vi "Drive to Distance.vi"(9 "Acceptable Error (in)":dbl, 10 "Target in Inches":dbl) -> (2 "Complete?":bool)   [LabVIEW 2020]
uses:
  Global Sensor Reads.vi
  <vilib>/Rock Robotics/WPI/RobotDrive/WPI_RobotDriveArcadeDrive_Standard(NoSaturation).vi
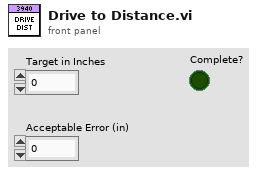
[diagram p1: front panel]
types:
  T1 = typedef "WPI_RobotDriveDevRef.ctl" = cluster{"DevStatus":errorcluster, "Motors[]":T2[], "Square Inputs":bool, "Max Output":dbl}
  T2 = typedef "WPI_MotorControlDeviceRef.ctl" = cluster{"DeviceStatus":errorcluster, "Type":T3, "PWM":cluster{"PWM Channel":T4, "DeadBand":T5}, "CAN":cluster{"Device Number":u8, "SetOutput VI Ref":variant, "GetOutput VI Ref":variant, "Enable VI Ref":variant, "Disable VI Ref":variant, "Data":variant}, "Invert":bool, "DIO PWM":cluster{"PWM \"Enable\" Channel":T4, "DIOChannel":T6, "PWM Rate":dbl}}
  T3 = typedef "WPI_MotorControlType.ctl" = enum16{"PWM", "CAN", "DIO PWM"}
  T4 = typedef "FPGA_DIOPWMChannel.ctl" = enum8{"PWM 0", "PWM 1", "PWM 2", "PWM 3", "PWM 4", "PWM 5", "PWM 6", "PWM 7", "PWM 8", "PWM 9", "PWM MXP 0", "PWM MXP 1", "PWM MXP 2", "PWM MXP 3", "PWM MXP 4", "PWM MXP 5", "PWM MXP 6", "PWM MXP 7", "PWM MXP 8", "PWM MXP 9", "Invalid"}
  T5 = typedef "WPI_PWMDeadband.ctl" = cluster{"Name":string, "maxPositivePwm":i32, "minPositivePwm":i32, "centerPwm":i32, "maxNegativePwm":i32, "minNegativePwm":i32, "angularRange":u16}
  T6 = typedef "FPGA_DIOChannel.ctl" = enum8{"DIO 0", "DIO 1", "DIO 2", "DIO 3", "DIO 4", "DIO 5", "DIO 6", "DIO 7", "DIO 8", "DIO 9", "DIO MXP 0", "DIO MXP 1", "DIO MXP 2", "DIO MXP 3", "DIO MXP 4", "DIO MXP 5", "DIO MXP 6", "DIO MXP 7", "DIO MXP 8", "DIO MXP 9", "DIO MXP 10", "DIO MXP 11", "DIO MXP 12", "DIO MXP 13", "DIO MXP 14", "DIO MXP 15", "SPI Port CS1", "SPI Port CS2", "SPI Port CS3", "SPI Port MISO", "SPI Port MOSI", "Invalid"}
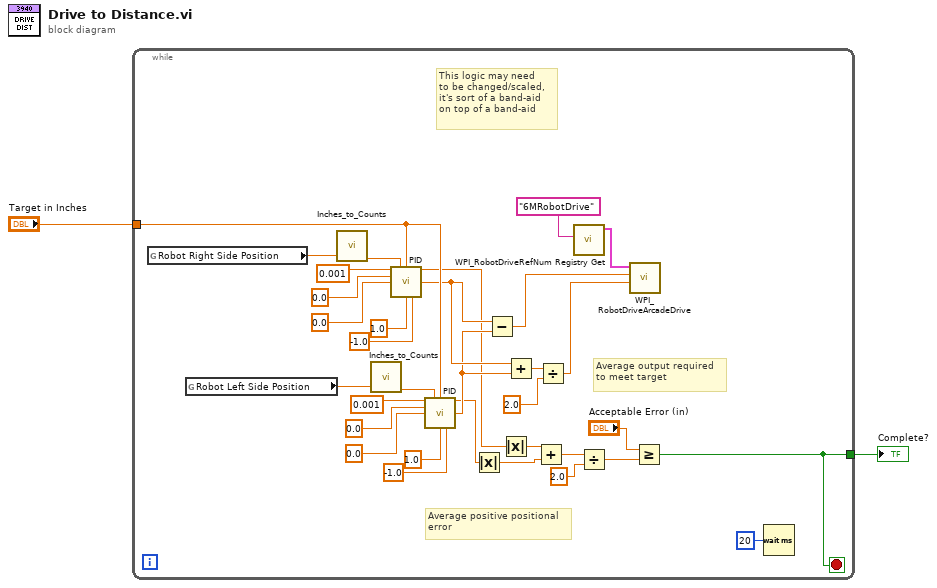
[diagram p0: block diagram]
diagram:
  n1 = while {
    tunnel: "Target in Inches" -> [w19]
    tunnel: [w4] -> w1
    stop <- w4 stop-if-true
    # "Average positive positional\nerror"
    # "Average output required\nto meet target"
    # "This logic may need\nto be changed/scaled,\nit's sort of a band-aid\non top of a band-aid"
    n2 = global read "Global Sensor Reads.vi" "Robot Right Side Position"() -> (w35:dbl)
    n3 = global read "Global Sensor Reads.vi" "Robot Left Side Position"() -> (w26:dbl)
    n4 = call "Inches_to_Counts.vi"("Encoder Counts Input"=w35) -> ("Inches Output"=w34:dbl)  [unwired: 9 in, 1 out]
    n5 = call "Inches_to_Counts.vi"("Encoder Counts Input"=w26) -> ("Inches Output"=w25:dbl)  [unwired: 9 in, 1 out]
    n6 = call "PID.vi"("Kp"=0.001, "Process Variable"=w34, "Goal"=w19, "Ki"=0.0, "Kd"=0.0, "Max Ouput"=1.0, "Min Output"=-1.0) -> ("Current Error"=w10:dbl, "Command"=w17:dbl)  [unwired: 6 in, 1 out]
    n7 = call "PID.vi"("Kp"=0.001, "Process Variable"=w25, "Goal"=w19, "Ki"=0.0, "Kd"=0.0, "Max Ouput"=1.0, "Min Output"=-1.0) -> ("Current Error"=w7:dbl, "Command"=w16:dbl)  [unwired: 6 in, 1 out]
    n8 = Absolute Value(x=w7) -> (abs(x)=w8:dbl)
    n9 = Subtract(x=w17, y=w16) -> (x-y=w18:dbl)
    n10 = Absolute Value(x=w10) -> (abs(x)=w9:dbl)
    n11 = Add(x=w17, y=w16) -> (x+y=w15:dbl)
    n12 = Add(x=w9, y=w8) -> (x+y=w11:dbl)
    n13 = Divide(x=w15, y=2.0) -> (x/y=w13:dbl)
    n14 = call <vilib>:"WPI_RobotDriveRefNum Registry Get.vi"("refnum name"="6MRobotDrive") -> ("RobotDriveDevRef"=w27:T1)  [unwired: 1 in, 9 out]
    n15 = Divide(x=w11, y=2.0) -> (x/y=w6:dbl)
    n16 = call-poly <vilib>:"WPI_RobotDriveArcadeDrive.vi"("Y axis value"=w13, "X axis value"=w18, "RobotDriveDevRef"=w27) -> ()  [unwired: 6 in, 3 out]
    n17 = Greater Or Equal?(x="Acceptable Error (in)", y=w6) -> (x >= y?=w4:bool)
    n18 = Wait (ms)(milliseconds to wait=u32 20) -> ()  [unwired: 1 out]
  }
  "Complete?" <- w1
